vi "Get Project Paths.vi"(7 "Flat Constructors?":bool, 8 "error in (no error)":errorcluster, 10 "Current Virtual Path":string, 11 "ProjectItem refnum":refnum<vi>) -> (0 "error out":errorcluster, 3 "Item Info":T1[](array[typedef]))   [LabVIEW 2023]
doc: "Gets paths on disk and virtual paths of each item contained within the project item identified by <B>ProjectItem Refnum</B>, taking into account its <B>Current Virtual Path</B>.\n\nThis VI is recursive."
uses:
  CTLs/Item Info.ctl
  <vilib>/Utility/libraryn.llb/Get File Extension.vi
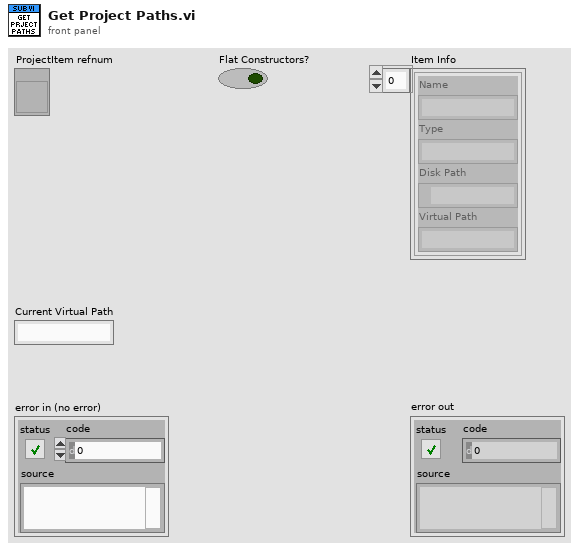
[diagram p1: front panel]
types:
  T1 = typedef "Item Info.ctl" = cluster{"Name":string, "Type":string, "Disk Path":path, "Virtual Path":string}
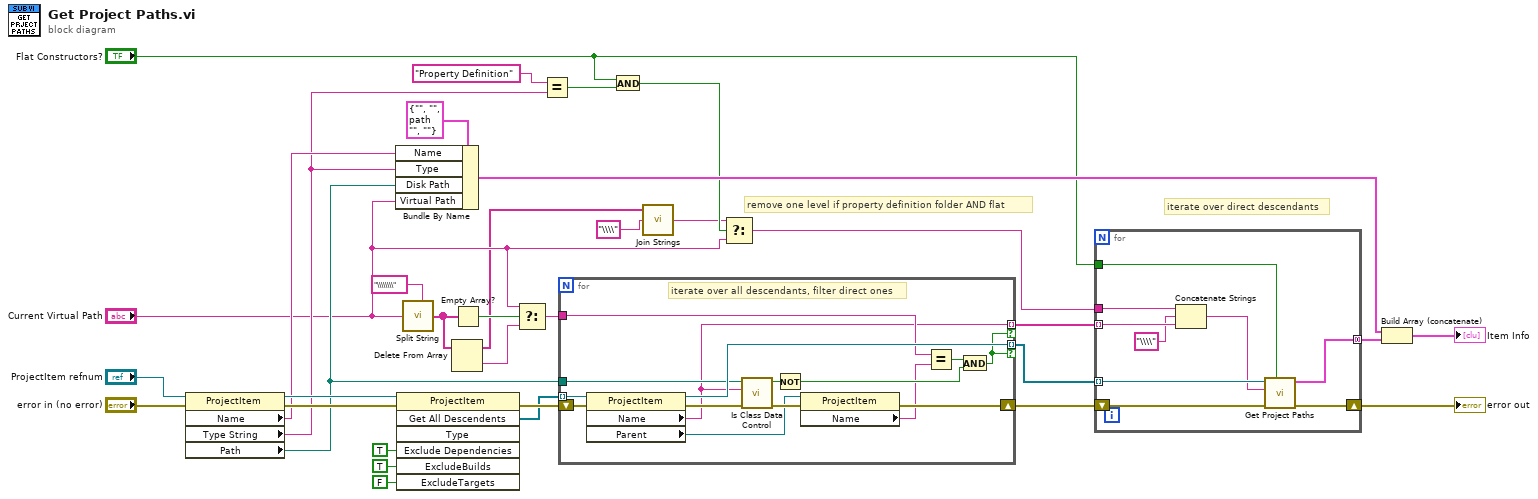
[diagram p0: block diagram]
diagram:
  # "remove one level if property definition folder AND flat"
  # "iterate over direct descendants"
  n1 = property class="ProjectItem"(reference="ProjectItem refnum", error in="error in (no error)") -> (reference out=w20:refnum<vi>, error out=w33:errorcluster, "Name"=w16:string, "Type String"=w11:string, "Path"=w15:path)
  n2 = Bundle By Name(cluster=T1 {"Name"="", "Type"="", "Disk Path"=path "", "Virtual Path"=""} ("Item Info"), "Name"=w16, "Type"=w11, "Disk Path"=w15, "Virtual Path"="Current Virtual Path") -> (w13:T1)
  n3 = invoke class="ProjectItem" method="Get All Descendents"(reference=w20, error in=w33, "Exclude Dependencies"=TRUE ("ExcludeDependencies"), "ExcludeBuilds"=TRUE, "ExcludeTargets"=FALSE) -> (error out=w34:errorcluster, "All Descendents"=w29:refnum<vi>[])  [unwired: 2 in, 5 out]
  n4 = call <vilib>:"Split String.vi"("Split Pattern"="\\\\\\\\", "Input String"="Current Virtual Path") -> ("Split String"=w7:string[])  [unwired: 5 in]
  n5 = Delete From Array(array=w7) -> (deleted portion=w22:string, array with subset deleted=w1:string[])  [unwired: 2 in]
  n6 = Empty Array?(array=w7) -> (empty?=w23:bool)
  n7 = Select(t="Current Virtual Path", s=w23, f=w22) -> (s? t:f=w21:string)
  n8 = Equal?(x="Property Definition", y=w11) -> (x = y?=w9:bool)
  n9 = for {
    tunnel: w29 -> [w45] mode=indexing
    tunnel: w21 -> [w42]
    tunnel: [w43] -> w26 mode=indexing if=w36
    tunnel: [w35] -> w25 mode=indexing if=w36
    shift-right: [w46] -> w31
    shift-left: w34 -> [w49]
    tunnel: w15 -> [w37]
    # "iterate over all descendants, filter direct ones"
    n10 = property class="ProjectItem"(reference=w45, error in=w49) -> (reference out=w43:refnum<vi>, error out=w48:errorcluster, "Name"=w35:string, "Parent"=w44:refnum<vi>)
    n11 = call "Is Class Data Control.vi"("error in (no error)"=w48, "Item Name"=w35, "Path"=w37) -> ("error out"=w47:errorcluster, "Is Class Data Control?"=w41:bool)  [unwired: 7 in]
    n12 = Not(x=w41) -> (.not. x?=w39:bool)
    n13 = property class="ProjectItem"(reference=w44, error in=w47) -> (error out=w46:errorcluster, "Name"=w38:string)  [unwired: 1 out]
    n14 = Equal?(x=w42, y=w38) -> (x = y?=w40:bool)
    n15 = And(x=w40, y=w39) -> (x .and. y?=w36:bool)
  }
  n16 = And(x="Flat Constructors?", y=w9) -> (x .and. y?=w5:bool)
  n17 = call <vilib>:"Join Strings.vi"("Separator (,)"="\\\\" ("Split Pattern"), "Strings In"=w1) -> ("String"=w4:string)  [unwired: 1 in]
  n18 = Select(t=w4, s=w5, f="Current Virtual Path") -> (s? t:f=w2:string)
  n19 = for {
    tunnel: w26 -> [w56] mode=indexing
    tunnel: w25 -> [w53] mode=indexing
    tunnel: w2 -> [w55]
    shift-right: [w57] -> w30
    shift-left: w31 -> [w58]
    tunnel: [w52] -> w14 mode=concatenating
    tunnel: "Flat Constructors?" -> [w51]
    n20 = Concatenate Strings(w55, "\\\\" ("string"), w53) -> (w54:string)
    n21 = call "Get Project Paths.vi"("Flat Constructors?"=w51, "error in (no error)"=w58, "Current Virtual Path"=w54, "ProjectItem refnum"=w56) -> ("error out"=w57:errorcluster, "Item Info"=w52:T1[])  [unwired: 6 in]
  }
  "error out" <- w30
  n22 = Build Array (concatenate)(w13, w14) -> (→"Item Info":T1[])
